vi "Init.vi"(8 "error in (no error)":errorcluster, 10 "PLC Settings":T1={"Port"="", "BaudRate"=9600, "Wakeup Signal Address "=0, "Acquisiton Address"=0, "Acknowledgement Address"=0, "Sleep Address"=0}, 11 "PLCHandler in":refnum<class "PLCHandler.lvclass">) -> (0 "error out":errorcluster, 3 "PLCHandler out":refnum<class "PLCHandler.lvclass">)   [LabVIEW 2022 SP3, in "PLCHandler.lvlib" / "PLCHandler.lvclass"]
uses:
  PLCHandler.lvclass
  Typedefs/PLC Settings.ctl
  PLCHandler.lvclass/PLCHandler.ctl
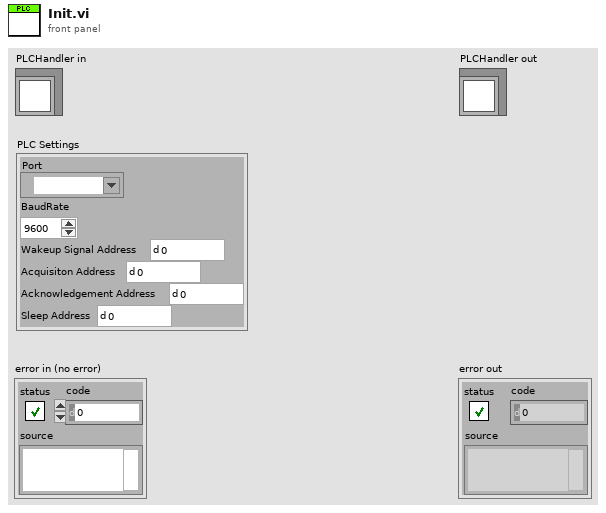
[diagram p1: front panel]
types:
  T1 = typedef "PLC Settings.ctl" = cluster{"Port":refnum<visa-resource-name>, "BaudRate":u32, "Wakeup Signal Address ":u16, "Acquisiton Address":u16, "Acknowledgement Address":u16, "Sleep Address":u16}
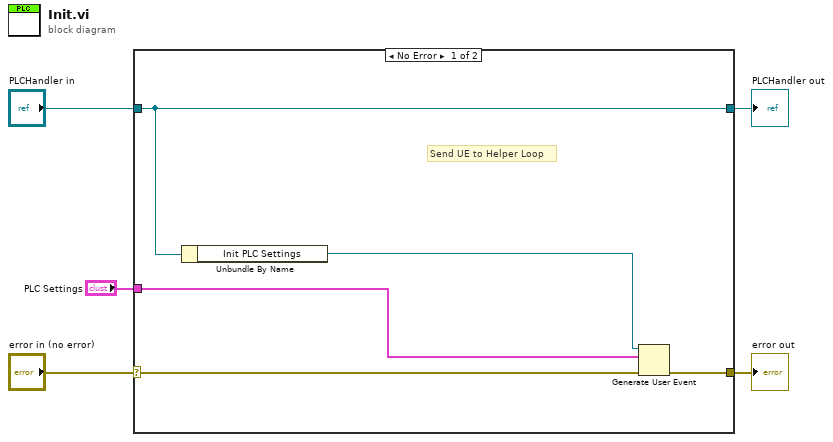
[diagram p0: block diagram]
diagram:
  n1 = case shown="No Error" "error in (no error)" {
    selector: "error in (no error)" -> [w7 w12]
    tunnel: [w10 w12] -> w4
    tunnel: [w8 w11] -> w2
    tunnel: "PLCHandler in" -> [w8 w11]
    tunnel: "PLC Settings" -> [w6 _]
    frame No Error {
      # "Send UE to Helper Loop"
      n2 = Unbundle By Name(w8) -> ("Init PLC Settings"=w9:refnum<user-event>)
      n3 = Generate User Event(user event=w9, event data cluster=w6, error in=w7) -> (error out=w10:errorcluster)  [unwired: 1 in, 1 out]
    }
    frame Error {
    }
  }
  "error out" <- w4
  "PLCHandler out" <- w2
